vi "Begin.vi"() -> (0 "CameraDevRef 2":T1, 1 "CameraDevRef":T1)   [LabVIEW 2011]
doc: "Called before other user functions, this VI is expected to open initial I/O refnums, load in file data, and do all program initialization. Notice that the <B>error out</B> terminal is simply used for data flow. Wiring it to other structures or subVIs ensures that this VI runs first."
uses:
  <vilib>/Rock Robotics/WPI/Camera/WPI_CameraDevRef.ctl
  <vilib>/Rock Robotics/SystemInterfaces/DIO/FPGA_DIOPWMChannel.ctl
  <vilib>/Rock Robotics/WPI/Joystick/WPI_JoystickDeviceEnum.ctl
  <vilib>/Rock Robotics/SystemInterfaces/AI/FPGA_AIChannel.ctl
  <vilib>/Rock Robotics/SystemInterfaces/DIO/FPGA_DIORelayChannel.ctl
  <vilib>/Rock Robotics/SystemInterfaces/DIO/FPGA_DIOChannel.ctl
  <vilib>/Rock Robotics/SystemInterfaces/AI/FPGA_AIGyroChannel.ctl
  <vilib>/Rock Robotics/WPI/Relay/WPI_RelayDirection.ctl
  <vilib>/Rock Robotics/WPI/Encoder/WPI_EncoderType.ctl
  <vilib>/Rock Robotics/WPI/DriverStation/DriverStationLCD/WPI_DriverStationLCDLCDLine.ctl
  <vilib>/Rock Robotics/WPI/MotorControl/WPI_MotorControlOpen Victor.vi
  <vilib>/Rock Robotics/WPI/MotorControl/WPI_MotorControlOpen Jaguar.vi
  Robot Global Data.vi
  <vilib>/Utility/file.llb/Read From Spreadsheet File (DBL).vi
  <vilib>/Rock Robotics/WPI/Counter/WPI_CounterDigitalInputToDigitalSource.vi
  <vilib>/Rock Robotics/SystemInterfaces/Typedef/FPGA_TypedefDigitalModule.ctl
  <vilib>/Rock Robotics/SystemInterfaces/Typedef/FPGA_TypedefAnalogModule.ctl
panel:
  out "Path and file":string
  in  "Balls In Robot At Start":dbl=2.0
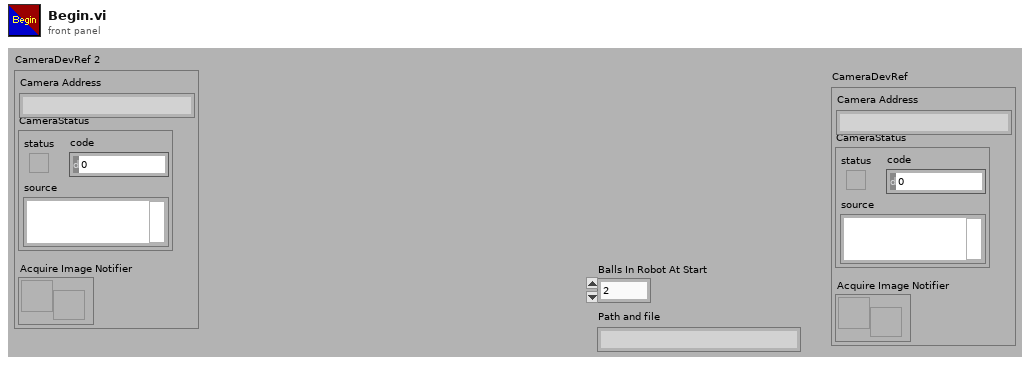
[diagram p1: front panel]
types:
  T1 = typedef "WPI_CameraDevRef.ctl" = cluster{"Camera Address":string, "CameraStatus":errorcluster, "Acquire Image Notifier":refnum<notifier>}
  T2 = typedef "WPI_DriverStationLCDLCDLine.ctl" = enum16{"Main - Line 1", "User - Line 2", "User - Line 3", "User - Line 4", "User - Line 5", "User - Line 6"}
  T3 = typedef "WPI_EncoderType.ctl" = enum16{"1x", "2x", "4x"}
  T4 = typedef "FPGA_DIOChannel.ctl" = enum8{"DIO 1", "DIO 2", "DIO 3", "DIO 4", "DIO 5", "DIO 6", "DIO 7", "DIO 8", "DIO 9", "DIO 10", "DIO 11", "DIO 12", "DIO 13", "DIO 14", "Invalid"}
  T5 = typedef "FPGA_DIORelayChannel.ctl" = enum8{"Relay 1", "Relay 2", "Relay 3", "Relay 4", "Relay 5", "Relay 6", "Relay 7", "Relay 8", "Invalid"}
  T6 = typedef "WPI_RelayDirection.ctl" = enum16{"Both directions", "Forward only", "Reverse only"}
  T7 = typedef "FPGA_AIGyroChannel.ctl" = enum8{"AI 1", "AI 2", "Invalid"}
  T8 = typedef "FPGA_DIOPWMChannel.ctl" = enum8{"PWM 1", "PWM 2", "PWM 3", "PWM 4", "PWM 5", "PWM 6", "PWM 7", "PWM 8", "PWM 9", "PWM 10", "Invalid"}
  T9 = typedef "FPGA_AIChannel.ctl" = enum8{"AI 1", "AI 2", "AI 3", "AI 4", "AI 5", "AI 6", "AI 7", "AI 8", "Invalid"}
  T10 = typedef "WPI_JoystickDeviceEnum.ctl" = enum16{"USB 1", "USB 2", "USB 3", "USB 4", "Kinect 1", "Kinect 2"}
  T11 = typedef "WPI_CameraImageSize.ctl" = enum16{"640x480", "320x240", "160x120"}
  T12 = cluster{"fps":i32, "compression":i32, "Image Size":T11}
  T13 = typedef "WPI_MotorControlDeviceRef.ctl" = cluster{"DeviceStatus":errorcluster, "Type":enum16{"PWM", "CAN"}, "PWM":cluster{"Digital Module":T14, "PWM Channel":T8, "DeadBand":T15}, "CAN":cluster{"Device Number":u8, "Control Mode":T16, "Semaphore":T17, "Max Vout":dbl}, "Invert":bool, "TransformRef":T18, "InvTransformRef":T18}
  T14 = typedef "FPGA_TypedefDigitalModule.ctl" = enum16{"Digital Module 1", "Digital Module 2"}
  T15 = typedef "WPI_PWMDeadband.ctl" = cluster{"Name":string, "maxPositivePwm":i32, "minPositivePwm":i32, "centerPwm":i32, "maxNegativePwm":i32, "minNegativePwm":i32, "angularRange":u16}
  T16 = typedef "WPI_CANJaguar_ControlMode.ctl" = enum8{"Percent VBus", "Current", "Speed", "Position", "Voltage"}
  T17 = typedef "Semaphore RefNum" = refnum<k1>
  T18 = typedef "WPI_PWMTransform_ConPane.ctl" = refnum<vi>
  T19 = typedef "WPI_ServoDeviceRef.ctl" = cluster{"DeviceStatus":errorcluster, "Digital Module":T14, "PWM Channel":T8, "DeadBand":T15}
  T20 = typedef "WPI_AnalogChannelDevRef.ctl" = cluster{"DevStatus":errorcluster, "Analog Module":T21, "Analog Channel":T9}
  T21 = typedef "FPGA_TypedefAnalogModule.ctl" = enum16{"Analog Module 1", "Analog Module 2"}
  T22 = typedef "WPI_CameraWhite Balance Values.ctl" = enum16{"Auto", "Fixed indoor", "Fixed outdoor 1", "Fixed outdoor 2", "Fixed fluorescent 1", "Fixed fluorescent 2", "Hold current"}
  T23 = typedef "WPI_JoystickDevRef.ctl" = cluster{"Device":T10}
  T24 = typedef "WPI_RelayDevRef.ctl" = cluster{"DevStatus":errorcluster, "Relay Channel":T5, "Digital Module":T14, "Relay Direction":T6}
  T25 = typedef "WPI_CameraExposure Values.ctl" = enum16{"Auto", "Flicker-free 50 Hz", "Flicker-free 60 Hz", "Hold current"}
  T26 = typedef "WPI_DigitalInputDevRef.ctl" = cluster{"DevStatus":errorcluster, "DIO Channel":T4, "Digital Module":T14}
  T27 = typedef "FPGA_CounterEncoderSourceConvertionLVSourceType.ctl" = cluster{"DevStatus":errorcluster, "AnalogTriggerMode?":bool, "DigitalMode":cluster{"Digital Module":T14, "DIO Channel":T28}, "AnalogTriggerMode":cluster{"AnalogTriggerIndex":T29, "OutputType":T30}}
  T28 = typedef "FPGA_DIODigitalSourceChannel.ctl" = enum8{"DIO 1", "DIO 2", "DIO 3", "DIO 4", "DIO 5", "DIO 6", "DIO 7", "DIO 8", "DIO 9", "DIO 10", "DIO 11", "DIO 12", "DIO 13", "DIO 14", "Disabled"}
  T29 = typedef "FPGA_AnalogTriggerIndex.ctl" = enum8{"Trig 0", "Trig 1", "Trig 2", "Trig 3", "Trig 4", "Trig 5", "Trig 6", "Trig 7", "Invalid"}
  T30 = typedef "FPGA_AnalogTriggerOutType.ctl" = enum16{"InWindow", "TriggerState", "Rising", "Falling"}
  T31 = typedef "WPI_EncoderDevRef.ctl" = cluster{"DevStatus":errorcluster, "EncoderIndex":T32, "CounterIndex":T33, "DistancePerCount":dbl, "Decoding Type":T3}
  T32 = typedef "FPGA_EncoderIdx.ctl" = enum8{"Enc 0", "Enc 1", "Enc 2", "Enc 3", "Invalid"}
  T33 = typedef "FPGA_CounterCtrSystemIndex.ctl" = enum8{"Ctr 0", "Ctr 1", "Ctr 2", "Ctr 3", "Ctr 4", "Ctr 5", "Ctr 6", "Ctr 7", "Invalid"}
  T34 = typedef "WPI_GyroDevRef.ctl" = cluster{"DevStatus":errorcluster, "Analog Module":T21, "Analog Channel":T9, "Offset":dbl, "Gain (VoltsPerDegree/Second)":dbl}
  T35 = typedef "WPI_UltrasonicDeviceRef.ctl" = cluster{"DevStatus":errorcluster, "Ping Digital Module":T14, "Echo Digital Module":T14, "Ping Channel":T4, "Echo Channel":T4, "CntIndex":T33}
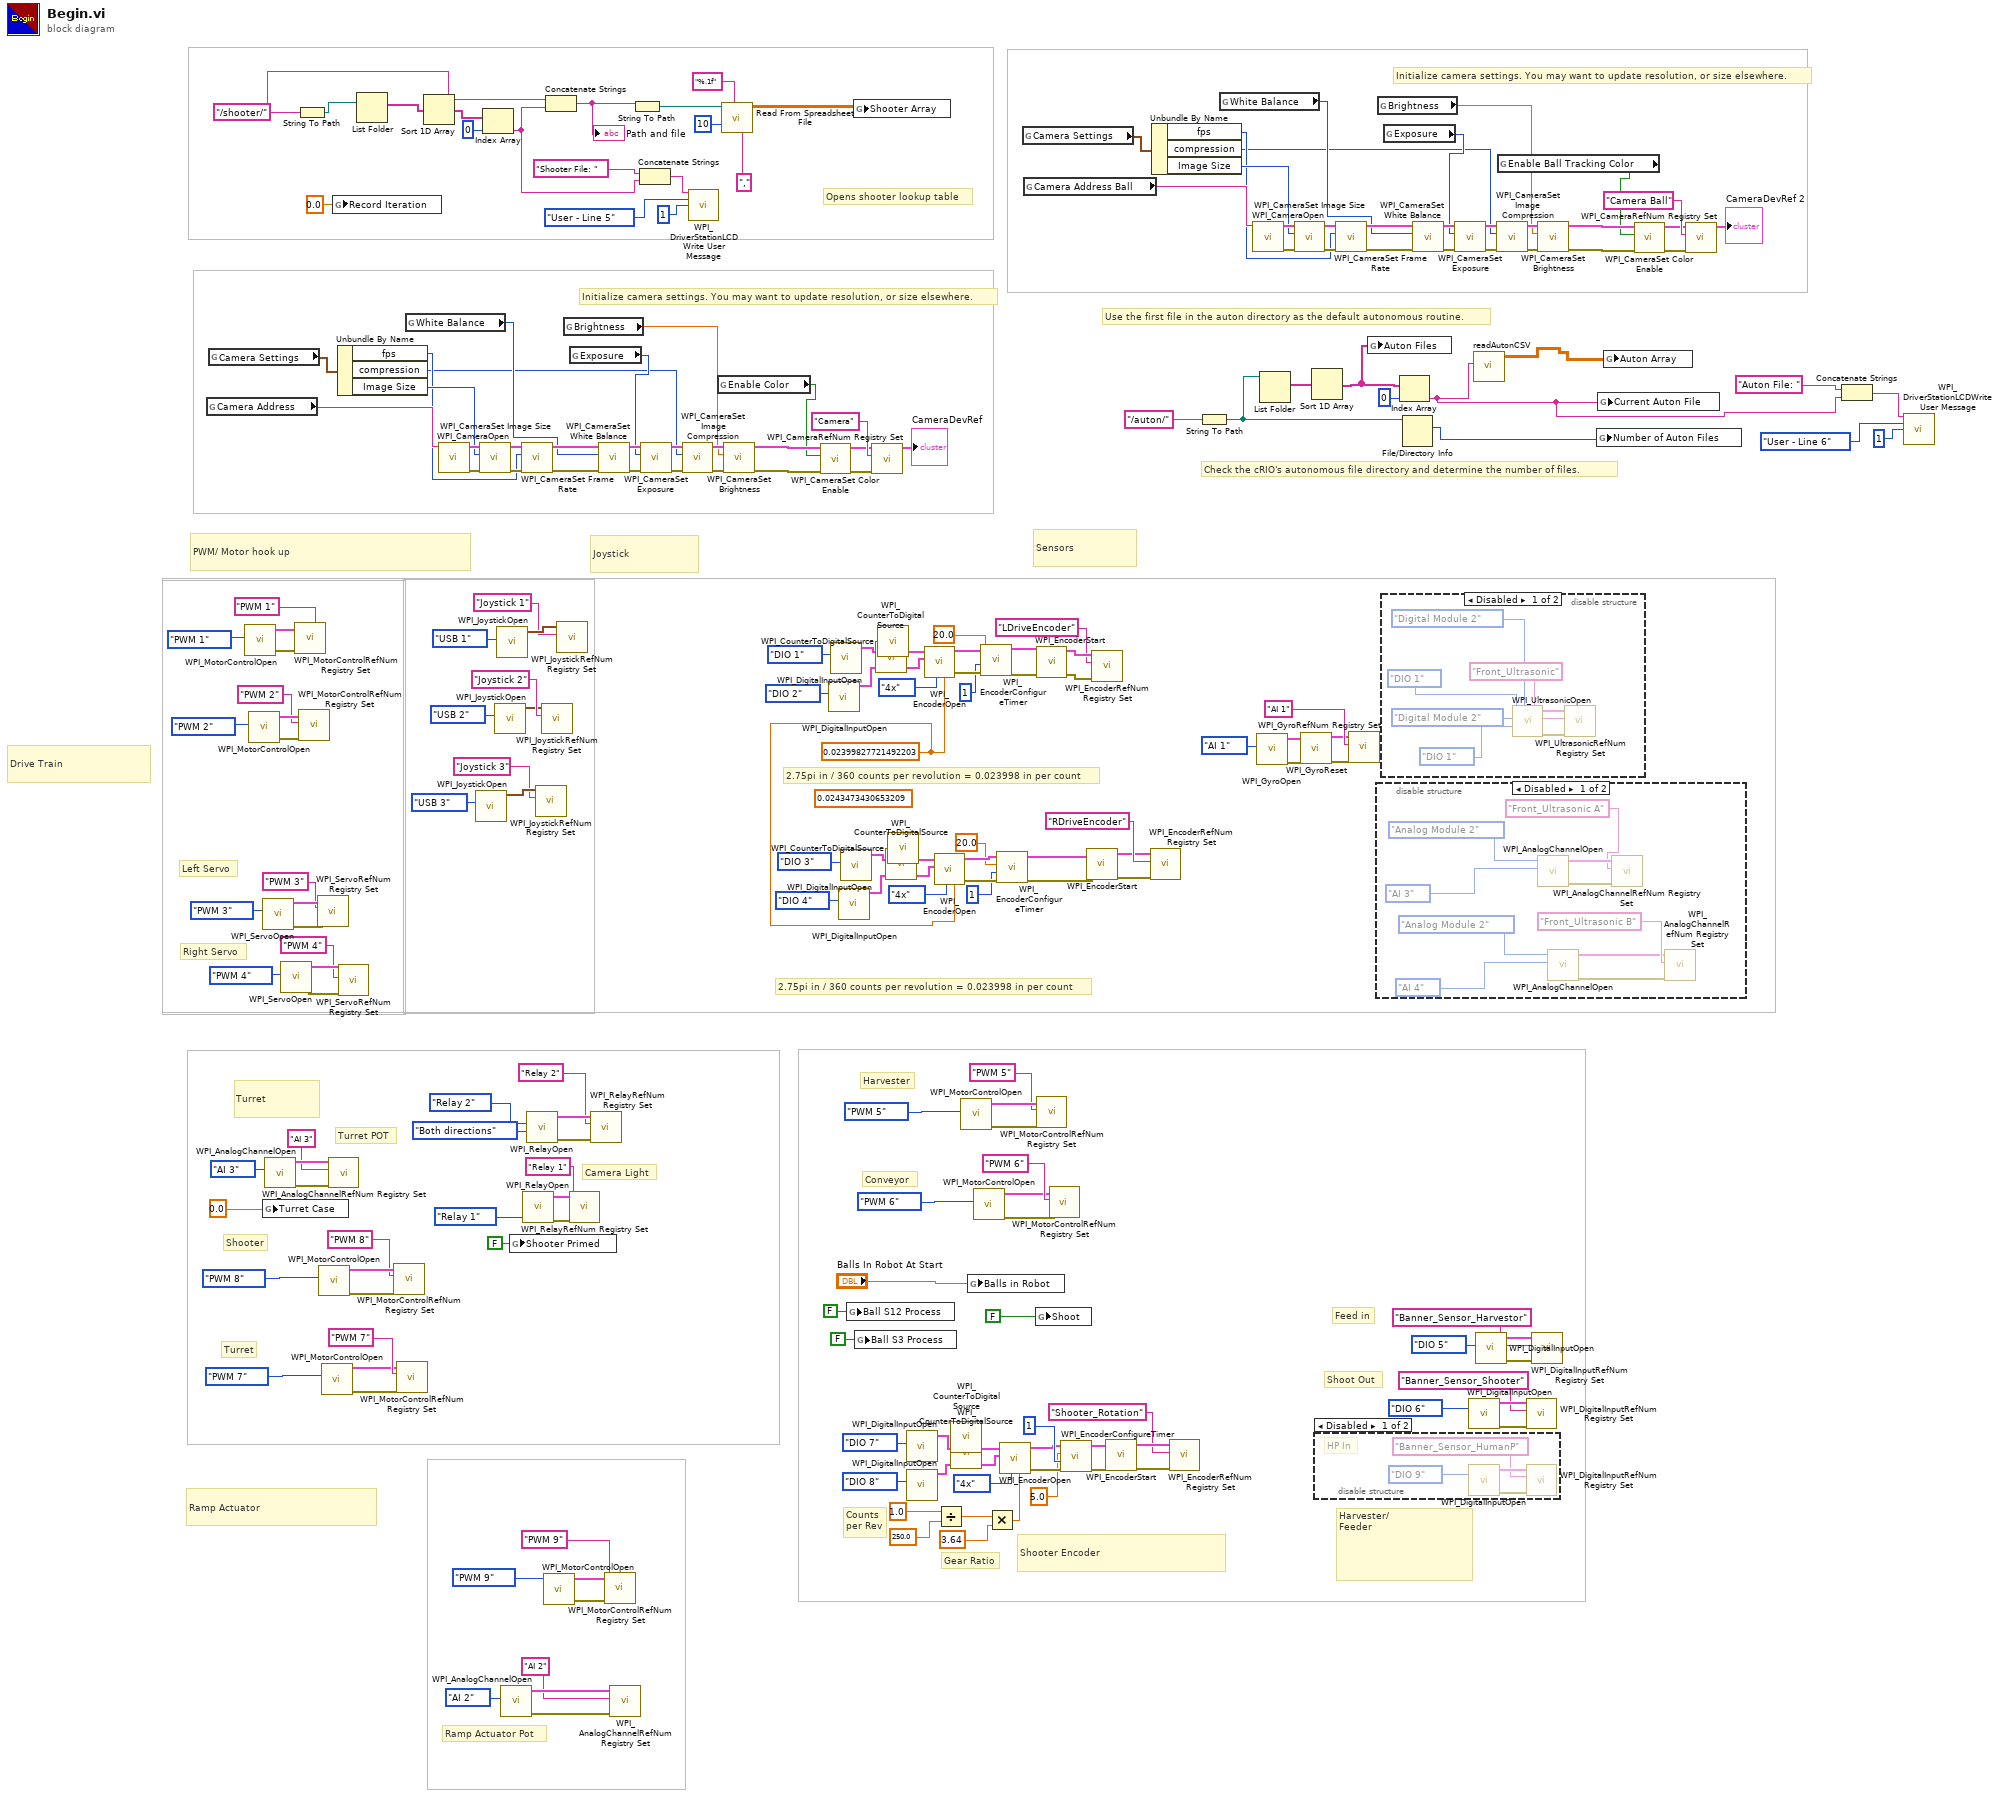
[diagram p0: block diagram]
diagram:
  (unwired) 0.0243473430653209 ("DistancePerCount")
  w59 = 0.02399827721492203 ("DistancePerCount")
  w107 = "/shooter/" ("string")
  # "Shooter Encoder"
  # "Counts\nper Rev"
  # "Gear Ratio"
  # "Initialize camera settings. You may want to update resolution, or size elsewhere."
  # "Check the cRIO's autonomous file directory and determine the number of files."
  # "Use the first file in the auton directory as the default autonomous routine."
  # "2.75pi in / 360 counts per revolution = 0.023998 in per count"
  # "2.75pi in / 360 counts per revolution = 0.023998 in per count"
  # "Opens shooter lookup table"
  # "Shoot Out"
  # "Feed in"
  # "Harvester"
  # "Conveyor"
  # "Shooter"
  # "Initialize camera settings. You may want to update resolution, or size elsewhere."
  # "Camera Light"
  # "Ramp Actuator Pot"
  # "Turret POT"
  # "Turret"
  # "Right Servo"
  # "Left Servo"
  # "Harvester/\nFeeder"
  # "Turret"
  # "Ramp Actuator"
  # "Drive Train"
  # "Sensors"
  # "Joystick"
  # "PWM/ Motor hook up"
  n1 = global read "Robot Global Data.vi" "Camera Address"() -> (w160:string)
  n2 = global read "Robot Global Data.vi" "Camera Settings"() -> (w159:T12)
  n3 = call-poly <vilib>:"WPI_MotorControlOpen.vi"("PWM Channel"=FPGA_DIOPWMChannel."PWM 1") -> ("error out"=w200:errorcluster, "MotorControlDeviceRef"=w202:T13)  [unwired: 9 in]
  n4 = call-poly <vilib>:"WPI_MotorControlOpen.vi"("PWM Channel"=FPGA_DIOPWMChannel."PWM 2") -> ("error out"=w198:errorcluster, "MotorControlDeviceRef"=w196:T13)  [unwired: 9 in]
  n5 = call <vilib>:"WPI_ServoOpen.vi"("PWM Channel"=FPGA_DIOPWMChannel."PWM 3") -> ("error out"=w213:errorcluster, "ServoDeviceRef"=w218:T19)  [unwired: 9 in]
  n6 = global write "Robot Global Data.vi" "Turret Case"(0.0 ("Return To Home Case")) -> ()
  n7 = call <vilib>:"WPI_AnalogChannelOpen.vi"("Analog Channel"=FPGA_AIChannel."AI 3") -> ("error out"=w189:errorcluster, "AIDeviceRef"=w190:T20)  [unwired: 9 in]
  n8 = call <vilib>:"WPI_ServoOpen.vi"("PWM Channel"=FPGA_DIOPWMChannel."PWM 4") -> ("error out"=w212:errorcluster, "ServoDeviceRef"=w216:T19)  [unwired: 9 in]
  n9 = call <vilib>:"WPI_MotorControlRefNum Registry Set.vi"("error in (no error)"=w200, "refnum name"="PWM 1", "MotorControlDevRef"=w202) -> ()  [unwired: 7 in, 2 out]
  n10 = String To Path(string=w107) -> (path=w116:path)
  n11 = call <vilib>:"WPI_MotorControlRefNum Registry Set.vi"("error in (no error)"=w198, "refnum name"="PWM 2", "MotorControlDevRef"=w196) -> ()  [unwired: 7 in, 2 out]
  n12 = call <vilib>:"WPI_ServoRefNum Registry Set.vi"("error in (no error)"=w213, "refnum name"="PWM 3", "ServoDeviceRef"=w218) -> ()  [unwired: 7 in, 2 out]
  n13 = call-poly <vilib>:"WPI_MotorControlOpen.vi"("PWM Channel"=FPGA_DIOPWMChannel."PWM 8") -> ("error out"=w143:errorcluster, "MotorControlDeviceRef"=w145:T13)  [unwired: 9 in]
  n14 = call-poly <vilib>:"WPI_MotorControlOpen.vi"("PWM Channel"=FPGA_DIOPWMChannel."PWM 7") -> ("error out"=w194:errorcluster, "MotorControlDeviceRef"=w192:T13)  [unwired: 9 in]
  n15 = call <vilib>:"WPI_AnalogChannelRefNum Registry Set.vi"("error in (no error)"=w189, "refnum name"="AI 3", "AIDeviceRef"=w190) -> ()  [unwired: 7 in, 2 out]
  n16 = global write "Robot Global Data.vi" "Record Iteration"(0.0 ("Record Iteration")) -> ()
  n17 = Unbundle By Name(w159) -> ("fps"=w157:i32, "compression"=w154:i32, "Image Size"=w158:T11)
  n18 = call <vilib>:"WPI_ServoRefNum Registry Set.vi"("error in (no error)"=w212, "refnum name"="PWM 4", "ServoDeviceRef"=w216) -> ()  [unwired: 7 in, 2 out]
  n19 = List Folder(path=w116) -> (filenames=w115:string[])  [unwired: 1 in, 5 out]
  n20 = call <vilib>:"WPI_MotorControlRefNum Registry Set.vi"("error in (no error)"=w143, "refnum name"="PWM 8", "MotorControlDevRef"=w145) -> ()  [unwired: 7 in, 2 out]
  n21 = call <vilib>:"WPI_MotorControlRefNum Registry Set.vi"("error in (no error)"=w194, "refnum name"="PWM 7", "MotorControlDevRef"=w192) -> ()  [unwired: 7 in, 2 out]
  n22 = global read "Robot Global Data.vi" "White Balance"() -> (w156:T22)
  n23 = Sort 1D Array(array=w115) -> (sorted array=w114:string[])
  n24 = call <vilib>:"WPI_CameraOpen.vi"("Camera Address"=w160) -> ("error out"=w166:errorcluster, "CameraDevRef"=w167:T1)  [unwired: 1 in, 8 out]
  n25 = call <vilib>:"WPI_JoystickOpen.vi"("JoystickDevice"=WPI_JoystickDeviceEnum."USB 3") -> ("JoystickDevRef"=w205:T23)  [unwired: 10 in]
  n26 = call <vilib>:"WPI_CameraSet Image Size.vi"("error in (no error)"=w166, "Image Size"=w158, "CameraDevRef"=w167) -> ("error out"=w165:errorcluster, "CameraDevRef Out"=w168:T1)  [unwired: 7 out]
  n27 = Index Array(array=w114, index=0) -> (element=w6:string)
  n28 = call <vilib>:"WPI_JoystickOpen.vi"("JoystickDevice"=WPI_JoystickDeviceEnum."USB 2") -> ("JoystickDevRef"=w208:T23)  [unwired: 10 in]
  n29 = call <vilib>:"WPI_JoystickOpen.vi"("JoystickDevice"=WPI_JoystickDeviceEnum."USB 1") -> ("JoystickDevRef"=w211:T23)  [unwired: 10 in]
  n30 = call <vilib>:"WPI_AnalogChannelOpen.vi"("Analog Channel"=FPGA_AIChannel."AI 2") -> ("error out"=w184:errorcluster, "AIDeviceRef"=w185:T20)  [unwired: 9 in]
  n31 = global write "Robot Global Data.vi" "Shooter Primed"(FALSE ("Ball S3 Process")) -> ()
  n32 = call <vilib>:"WPI_CameraSet Frame Rate.vi"("error in (no error)"=w165, "Frame Rate (fps)"=w157, "CameraDevRef"=w168) -> ("error out"=w164:errorcluster, "CameraDevRef Out"=w170:T1)  [unwired: 7 out]
  n33 = call <vilib>:"WPI_RelayOpen.vi"("Relay Channel"=FPGA_DIORelayChannel."Relay 1") -> ("error out"=w177:errorcluster, "RelayDevRef"=w176:T24)  [unwired: 9 in]
  n34 = call <vilib>:"WPI_RelayOpen.vi"("Relay Direction"=WPI_RelayDirection."Both directions", "Relay Channel"=FPGA_DIORelayChannel."Relay 2") -> ("error out"=w102:errorcluster, "RelayDevRef"=w103:T24)  [unwired: 8 in]
  n35 = call <vilib>:"WPI_JoystickRefNum Registry Set.vi"("refnum name"="Joystick 3", "JoystickDevRef"=w205) -> ()  [unwired: 8 in, 2 out]
  n36 = call <vilib>:"WPI_JoystickRefNum Registry Set.vi"("refnum name"="Joystick 2", "JoystickDevRef"=w208) -> ()  [unwired: 8 in, 2 out]
  n37 = call-poly <vilib>:"WPI_MotorControlOpen.vi"("PWM Channel"=FPGA_DIOPWMChannel."PWM 9") -> ("error out"=w180:errorcluster, "MotorControlDeviceRef"=w181:T13)  [unwired: 9 in]
  n38 = Concatenate Strings(w107, w6) -> (w109:string)
  "Path and file" <- w109
  n39 = call <vilib>:"WPI_JoystickRefNum Registry Set.vi"("refnum name"="Joystick 1", "JoystickDevRef"=w211) -> ()  [unwired: 8 in, 2 out]
  n40 = global read "Robot Global Data.vi" "Brightness"() -> (w153:dbl)
  n41 = global read "Robot Global Data.vi" "Exposure"() -> (w155:T25)
  n42 = call <vilib>:"WPI_RelayRefNum Registry Set.vi"("error in (no error)"=w177, "refnum name"="Relay 1", "RelayDevRef"=w176) -> ()  [unwired: 7 in, 2 out]
  n43 = call <vilib>:"WPI_RelayRefNum Registry Set.vi"("error in (no error)"=w102, "refnum name"="Relay 2", "RelayDevRef"=w103) -> ()  [unwired: 7 in, 2 out]
  n44 = call <vilib>:"WPI_CameraSet White Balance.vi"("error in (no error)"=w164, "White Balance"=w156, "CameraDevRef"=w170) -> ("error out"=w163:errorcluster, "CameraDevRef Out"=w169:T1)  [unwired: 7 out]
  n45 = call <vilib>:"WPI_MotorControlRefNum Registry Set.vi"("error in (no error)"=w180, "refnum name"="PWM 9", "MotorControlDevRef"=w181) -> ()  [unwired: 7 in, 2 out]
  n46 = call <vilib>:"WPI_AnalogChannelRefNum Registry Set.vi"("error in (no error)"=w184, "refnum name"="AI 2", "AIDeviceRef"=w185) -> ()  [unwired: 7 in, 2 out]
  n47 = String To Path(string=w109) -> (path=w108:path)
  n48 = Concatenate Strings("Shooter File: ", w6) -> (w4:string)
  n49 = call <vilib>:"WPI_CameraSet Exposure.vi"("error in (no error)"=w163, "Exposure"=w155, "CameraDevRef"=w169) -> ("error out"=w162:errorcluster, "CameraDevRef Out"=w172:T1)  [unwired: 7 out]
  n50 = call <vilib>:"WPI_CameraSet Image Compression.vi"("error in (no error)"=w162, "Compression"=w154, "CameraDevRef"=w172) -> ("error out"=w161:errorcluster, "CameraDevRef Out"=w171:T1)  [unwired: 7 out]
  n51 = call <vilib>:"WPI_DriverStationLCDWrite User Message.vi"("line text"=w4, "line"=WPI_DriverStationLCDLCDLine."User - Line 5", "starting column"=i8 1) -> ()  [unwired: 2 in, 11 out]
  n52 = global read "Robot Global Data.vi" "Enable Color"() -> (w148:bool)
  n53 = call-poly <vilib>:"Read From Spreadsheet File.vi"("delimiter (\\t)"="," ("delimiter (\\t)"), "format (%.3f)"="%.1f", "number of rows (all:-1)"=10, "file path (dialog if empty)"=w108) -> ("all rows"=w106:dbl[][])  [unwired: 1 in, 6 out]
  n54 = call <vilib>:"WPI_CameraSet Brightness.vi"("error in (no error)"=w161, "Brightness"=w153, "CameraDevRef"=w171) -> ("error out"=w151:errorcluster, "CameraDevRef Out"=w152:T1)  [unwired: 7 out]
  n55 = call <vilib>:"WPI_CameraSet Color Enable.vi"("error in (no error)"=w151, "Color Enabled"=w148, "CameraDevRef"=w152) -> ("error out"=w149:errorcluster, "CameraDevRef Out"=w150:T1)  [unwired: 7 in]
  n56 = call <vilib>:"WPI_DigitalInputOpen.vi"("DIO Channel"=FPGA_DIOChannel."DIO 2") -> ("DigitalInputDevRef"=w94:T26)  [unwired: 9 in, 1 out]
  n57 = call <vilib>:"WPI_DigitalInputOpen.vi"("DIO Channel"=FPGA_DIOChannel."DIO 1") -> ("DigitalInputDevRef"=w91:T26)  [unwired: 9 in, 1 out]
  n58 = call <vilib>:"WPI_DigitalInputOpen.vi"("DIO Channel"=FPGA_DIOChannel."DIO 4") -> ("DigitalInputDevRef"=w85:T26)  [unwired: 9 in, 1 out]
  n59 = call <vilib>:"WPI_DigitalInputOpen.vi"("DIO Channel"=FPGA_DIOChannel."DIO 3") -> ("DigitalInputDevRef"=w88:T26)  [unwired: 9 in, 1 out]
  n60 = global write "Robot Global Data.vi" "Ball S12 Process"(FALSE ("Ball S12 Process")) -> ()
  n61 = global write "Robot Global Data.vi" "Shooter Array"(w106) -> ()
  n62 = global write "Robot Global Data.vi" "Ball S3 Process"(FALSE ("Ball S3 Process")) -> ()
  n63 = call <vilib>:"WPI_CameraRefNum Registry Set.vi"("error in (no error)"=w149, "refnum name"="Camera", "CameraDevRef"=w150) -> ("CameraDevRef"=→"CameraDevRef":T1)  [unwired: 8 out]
  n64 = call-poly <vilib>:"WPI_CounterToDigitalSource.vi"("DigitalInputDevRef"=w94) -> ("Digital Source"=w95:T27)  [unwired: 6 in]
  n65 = call-poly <vilib>:"WPI_CounterToDigitalSource.vi"("DigitalInputDevRef"=w91) -> ("Digital Source"=w90:T27)  [unwired: 6 in]
  n66 = call-poly <vilib>:"WPI_CounterToDigitalSource.vi"("DigitalInputDevRef"=w85) -> ("Digital Source"=w84:T27)  [unwired: 6 in]
  n67 = call-poly <vilib>:"WPI_CounterToDigitalSource.vi"("DigitalInputDevRef"=w88) -> ("Digital Source"=w89:T27)  [unwired: 6 in]
  n68 = call <vilib>:"WPI_DigitalInputOpen.vi"("DIO Channel"=FPGA_DIOChannel."DIO 7") -> ("DigitalInputDevRef"=w43:T26)  [unwired: 9 in, 1 out]
  n69 = call <vilib>:"WPI_DigitalInputOpen.vi"("DIO Channel"=FPGA_DIOChannel."DIO 8") -> ("DigitalInputDevRef"=w46:T26)  [unwired: 9 in, 1 out]
  n70 = call <vilib>:"WPI_EncoderOpen.vi"("DistancePerCount"=w59, "Decoding Type"=WPI_EncoderType."4x", "BSource"=w95, "ASource"=w90) -> ("error out"=w63:errorcluster, "EncoderDevRef"=w66:T31)  [unwired: 6 in]
  n71 = call <vilib>:"WPI_EncoderOpen.vi"("DistancePerCount"=w59, "Decoding Type"=WPI_EncoderType."4x", "BSource"=w84, "ASource"=w89) -> ("error out"=w81:errorcluster, "EncoderDevRef"=w80:T31)  [unwired: 6 in]
  n72 = Divide(x=1.0, y=250.0) -> (x/y=w40:dbl)
  n73 = call-poly <vilib>:"WPI_CounterToDigitalSource.vi"("DigitalInputDevRef"=w43) -> ("Digital Source"=w42:T27)  [unwired: 6 in]
  n74 = call-poly <vilib>:"WPI_CounterToDigitalSource.vi"("DigitalInputDevRef"=w46) -> ("Digital Source"=w47:T27)  [unwired: 6 in]
  n75 = call-poly <vilib>:"WPI_MotorControlOpen.vi"("PWM Channel"=FPGA_DIOPWMChannel."PWM 5") -> ("error out"=w139:errorcluster, "MotorControlDeviceRef"=w141:T13)  [unwired: 9 in]
  n76 = global write "Robot Global Data.vi" "Balls in Robot"("Balls In Robot At Start") -> ()
  n77 = call-poly <vilib>:"WPI_MotorControlOpen.vi"("PWM Channel"=FPGA_DIOPWMChannel."PWM 6") -> ("error out"=w138:errorcluster, "MotorControlDeviceRef"=w136:T13)  [unwired: 9 in]
  n78 = call <vilib>:"WPI_EncoderConfigureTimer.vi"("error in (no error)"=w63, "Number Samples to Average"=u8 1, "Minimum Rate"=20.0, "EncoderDevRef"=w66) -> ("error out"=w64:errorcluster, "EncoderDevRef"=w65:T31)  [unwired: 6 in]
  n79 = Multiply(x=w40, y=3.64) -> (x*y=w38:dbl)
  n80 = call <vilib>:"WPI_EncoderConfigureTimer.vi"("error in (no error)"=w81, "Number Samples to Average"=u8 1, "Minimum Rate"=20.0, "EncoderDevRef"=w80) -> ("error out"=w77:errorcluster, "EncoderDevRef"=w78:T31)  [unwired: 6 in]
  n81 = call <vilib>:"WPI_EncoderOpen.vi"("DistancePerCount"=w38, "Decoding Type"=WPI_EncoderType."4x", "BSource"=w47, "ASource"=w42) -> ("error out"=w50:errorcluster, "EncoderDevRef"=w51:T31)  [unwired: 6 in]
  n82 = global read "Robot Global Data.vi" "Camera Settings"() -> (w23:T12)
  n83 = global read "Robot Global Data.vi" "Camera Address Ball"() -> (w24:string)
  n84 = global write "Robot Global Data.vi" "Shoot"(FALSE ("Ball S12 Process")) -> ()
  n85 = call <vilib>:"WPI_EncoderStart.vi"("error in (no error)"=w64, "EncoderDevRef"=w65) -> ("error out"=w98:errorcluster, "EncoderDevRef"=w97:T31)  [unwired: 8 in]
  n86 = call <vilib>:"WPI_MotorControlRefNum Registry Set.vi"("error in (no error)"=w139, "refnum name"="PWM 5", "MotorControlDevRef"=w141) -> ()  [unwired: 7 in, 2 out]
  n87 = call <vilib>:"WPI_MotorControlRefNum Registry Set.vi"("error in (no error)"=w138, "refnum name"="PWM 6", "MotorControlDevRef"=w136) -> ()  [unwired: 7 in, 2 out]
  n88 = call <vilib>:"WPI_EncoderConfigureTimer.vi"("error in (no error)"=w50, "Number Samples to Average"=u8 1, "Minimum Rate"=5.0, "EncoderDevRef"=w51) -> ("error out"=w54:errorcluster, "EncoderDevRef"=w53:T31)  [unwired: 6 in]
  n89 = call <vilib>:"WPI_EncoderStart.vi"("error in (no error)"=w77, "EncoderDevRef"=w78) -> ("error out"=w75:errorcluster, "EncoderDevRef"=w76:T31)  [unwired: 8 in]
  n90 = call <vilib>:"WPI_EncoderRefNum Registry Set.vi"("error in (no error)"=w98, "refnum name"="LDriveEncoder", "EncoderDevRef"=w97) -> ()  [unwired: 7 in, 2 out]
  n91 = call <vilib>:"WPI_EncoderStart.vi"("error in (no error)"=w54, "EncoderDevRef"=w53) -> ("error out"=w56:errorcluster, "EncoderDevRef"=w55:T31)  [unwired: 8 in]
  n92 = call <vilib>:"WPI_EncoderRefNum Registry Set.vi"("error in (no error)"=w75, "refnum name"="RDriveEncoder", "EncoderDevRef"=w76) -> ()  [unwired: 7 in, 2 out]
  n93 = Unbundle By Name(w23) -> ("fps"=w21:i32, "compression"=w18:i32, "Image Size"=w22:T11)
  n94 = call <vilib>:"WPI_EncoderRefNum Registry Set.vi"("error in (no error)"=w56, "refnum name"="Shooter_Rotation", "EncoderDevRef"=w55) -> ()  [unwired: 7 in, 2 out]
  n95 = String To Path(string="/auton/") -> (path=w71:path)
  n96 = global read "Robot Global Data.vi" "White Balance"() -> (w20:T22)
  n97 = call <vilib>:"WPI_CameraOpen.vi"("Camera Address"=w24) -> ("error out"=w30:errorcluster, "CameraDevRef"=w31:T1)  [unwired: 1 in, 8 out]
  n98 = call <vilib>:"WPI_GyroOpen.vi"("Analog Channel"=FPGA_AIGyroChannel."AI 1") -> ("error out"=w119:errorcluster, "GyroDevRef"=w120:T34)  [unwired: 8 in, 1 out]
  n99 = List Folder(path=w71) -> (filenames=w70:string[])  [unwired: 1 in, 5 out]
  n100 = call <vilib>:"WPI_CameraSet Image Size.vi"("error in (no error)"=w30, "Image Size"=w22, "CameraDevRef"=w31) -> ("error out"=w29:errorcluster, "CameraDevRef Out"=w32:T1)  [unwired: 7 out]
  n101 = call <vilib>:"WPI_GyroReset.vi"("error in (no error)"=w119, "GyroDevRef"=w120) -> ("error out"=w118:errorcluster, "GyroDevRef"=w117:T34)  [unwired: 8 in]
  n102 = Sort 1D Array(array=w70) -> (sorted array=w68:string[])
  n103 = disable-structure shown="Disabled" {
    frame Disabled {
      # "HP In"
      n104 = call <vilib>:"WPI_DigitalInputOpen.vi"("DIO Channel"=FPGA_DIOChannel."DIO 9") -> ("error out"=w222:errorcluster, "DigitalInputDevRef"=w221:T26)  [unwired: 9 in]
      n105 = call <vilib>:"WPI_DigitalInputRefNum Registry Set.vi"("error in (no error)"=w222, "refnum name"="Banner_Sensor_HumanP", "DigitalInputDevRef"=w221) -> ()  [unwired: 7 in, 2 out]
    }
    frame Enabled {
    }
  }
  n106 = call <vilib>:"WPI_CameraSet Frame Rate.vi"("error in (no error)"=w29, "Frame Rate (fps)"=w21, "CameraDevRef"=w32) -> ("error out"=w28:errorcluster, "CameraDevRef Out"=w34:T1)  [unwired: 7 out]
  n107 = call <vilib>:"WPI_GyroRefNum Registry Set.vi"("error in (no error)"=w118, "refnum name"="AI 1", "GyroDevRef"=w117) -> ()  [unwired: 7 in, 2 out]
  n108 = global write "Robot Global Data.vi" "Auton Files"(w68) -> ()
  n109 = disable-structure shown="Disabled" {
    frame Disabled {
      n110 = call <vilib>:"WPI_AnalogChannelOpen.vi"("Analog Channel"=FPGA_AIChannel."AI 3", "Analog Module (Module 1)"=FPGA_TypedefAnalogModule."Analog Module 2") -> ("error out"=w229:errorcluster, "AIDeviceRef"=w228:T20)  [unwired: 8 in]
      n111 = call <vilib>:"WPI_AnalogChannelOpen.vi"("Analog Channel"=FPGA_AIChannel."AI 4", "Analog Module (Module 1)"=FPGA_TypedefAnalogModule."Analog Module 2") -> ("error out"=w224:errorcluster, "AIDeviceRef"=w225:T20)  [unwired: 8 in]
      n112 = call <vilib>:"WPI_AnalogChannelRefNum Registry Set.vi"("error in (no error)"=w229, "refnum name"="Front_Ultrasonic A", "AIDeviceRef"=w228) -> ()  [unwired: 7 in, 2 out]
      n113 = call <vilib>:"WPI_AnalogChannelRefNum Registry Set.vi"("error in (no error)"=w224, "refnum name"="Front_Ultrasonic B", "AIDeviceRef"=w225) -> ()  [unwired: 7 in, 2 out]
    }
    frame Enabled {
    }
  }
  n114 = global read "Robot Global Data.vi" "Brightness"() -> (w17:dbl)
  n115 = disable-structure shown="Disabled" {
    frame Disabled {
      n116 = call <vilib>:"WPI_UltrasonicOpen.vi"("Ping Digital Module (Module 1)"=FPGA_TypedefDigitalModule."Digital Module 2", "Echo DIO Channel"=FPGA_DIOChannel."DIO 1", "Echo Digital Module (Module 1)"=FPGA_TypedefDigitalModule."Digital Module 2", "Ping DIO Channel"=FPGA_DIOChannel."DIO 1") -> ("error out"=w240:errorcluster, "UltrasonicDevRef"=w239:T35)  [unwired: 6 in]
      n117 = call <vilib>:"WPI_UltrasonicRefNum Registry Set.vi"("error in (no error)"=w240, "refnum name"="Front_Ultrasonic", "UltrasonicDevRef"=w239) -> ()  [unwired: 7 in, 2 out]
    }
    frame Enabled {
    }
  }
  n118 = global read "Robot Global Data.vi" "Exposure"() -> (w19:T25)
  n119 = Index Array(array=w68, index=0) -> (element=w2:string)
  n120 = File/Directory Info(path=w71) -> (size=w73:i64)  [unwired: 1 in, 6 out]
  n121 = call <vilib>:"WPI_CameraSet White Balance.vi"("error in (no error)"=w28, "White Balance"=w20, "CameraDevRef"=w34) -> ("error out"=w27:errorcluster, "CameraDevRef Out"=w33:T1)  [unwired: 7 out]
  n122 = call <vilib>:"WPI_CameraSet Exposure.vi"("error in (no error)"=w27, "Exposure"=w19, "CameraDevRef"=w33) -> ("error out"=w26:errorcluster, "CameraDevRef Out"=w36:T1)  [unwired: 7 out]
  n123 = call <vilib>:"WPI_DigitalInputOpen.vi"("DIO Channel"=FPGA_DIOChannel."DIO 6") -> ("error out"=w129:errorcluster, "DigitalInputDevRef"=w128:T26)  [unwired: 9 in]
  n124 = call "readAutonCSV.vi"("AutonFile"=w2) -> ("AutonArray"=w67:dbl[][])  [unwired: 7 in]
  n125 = call <vilib>:"WPI_DigitalInputOpen.vi"("DIO Channel"=FPGA_DIOChannel."DIO 5") -> ("error out"=w132:errorcluster, "DigitalInputDevRef"=w131:T26)  [unwired: 9 in]
  n126 = call <vilib>:"WPI_CameraSet Image Compression.vi"("error in (no error)"=w26, "Compression"=w18, "CameraDevRef"=w36) -> ("error out"=w25:errorcluster, "CameraDevRef Out"=w35:T1)  [unwired: 7 out]
  n127 = global read "Robot Global Data.vi" "Enable Ball Tracking Color"() -> (w12:bool)
  n128 = call <vilib>:"WPI_DigitalInputRefNum Registry Set.vi"("error in (no error)"=w129, "refnum name"="Banner_Sensor_Shooter", "DigitalInputDevRef"=w128) -> ()  [unwired: 7 in, 2 out]
  n129 = call <vilib>:"WPI_DigitalInputRefNum Registry Set.vi"("error in (no error)"=w132, "refnum name"="Banner_Sensor_Harvestor", "DigitalInputDevRef"=w131) -> ()  [unwired: 7 in, 2 out]
  n130 = call <vilib>:"WPI_CameraSet Brightness.vi"("error in (no error)"=w25, "Brightness"=w17, "CameraDevRef"=w35) -> ("error out"=w15:errorcluster, "CameraDevRef Out"=w16:T1)  [unwired: 7 out]
  n131 = global write "Robot Global Data.vi" "Number of Auton Files"(w73) -> ()
  n132 = global write "Robot Global Data.vi" "Current Auton File"(w2) -> ()
  n133 = global write "Robot Global Data.vi" "Auton Array"(w67) -> ()
  n134 = call <vilib>:"WPI_CameraSet Color Enable.vi"("error in (no error)"=w15, "Color Enabled"=w12, "CameraDevRef"=w16) -> ("error out"=w13:errorcluster, "CameraDevRef Out"=w14:T1)  [unwired: 7 in]
  n135 = call <vilib>:"WPI_CameraRefNum Registry Set.vi"("error in (no error)"=w13, "refnum name"="Camera Ball", "CameraDevRef"=w14) -> ("CameraDevRef"=→"CameraDevRef 2":T1)  [unwired: 8 out]
  n136 = Concatenate Strings("Auton File: ", w2) -> (w1:string)
  n137 = call <vilib>:"WPI_DriverStationLCDWrite User Message.vi"("line text"=w1, "line"=WPI_DriverStationLCDLCDLine."User - Line 6", "starting column"=i8 1) -> ()  [unwired: 2 in, 11 out]
